vi "Configure Modulation(ASK).vi"(0 "VISA resource name":refnum<visa-resource-name>, 1 "Enable ASK Modulation (F: Disable)":bool, 2 "ASK Amplitude (0 Vpp)":dbl, 5 "Channel (1: Channel 1)":i32(ring)=1 items=["Channel 1"=1, "Channel 2"=2], 7 "ASK Source (0: Internal)":i32(ring) items=["Internal", "External"], 9 "Modulating Polarity (0: Positive)":i32(ring) items=["Positive", "Negative"], 11 "error in (no error)":errorcluster, 12 "Amplitude Unit (0: Vpp)":i32(ring) items=["Vpp", "Vrms", "dBm"], 13 "ASK Rate (100 Hz)":dbl=100.0) -> (4 "VISA resource name out":refnum<visa-resource-name>, 15 "error out":errorcluster)   [LabVIEW 2012, in "RIGOL DG4000 Series.lvlib"]
doc: "Configures ASK (Amplitude Shift Keying) modulation."
uses:
  <instrlib>/RIGOL DG4000 Series/RIGOL DG4000 Series.lvlib
panel:
  # "Amplitude Settings"
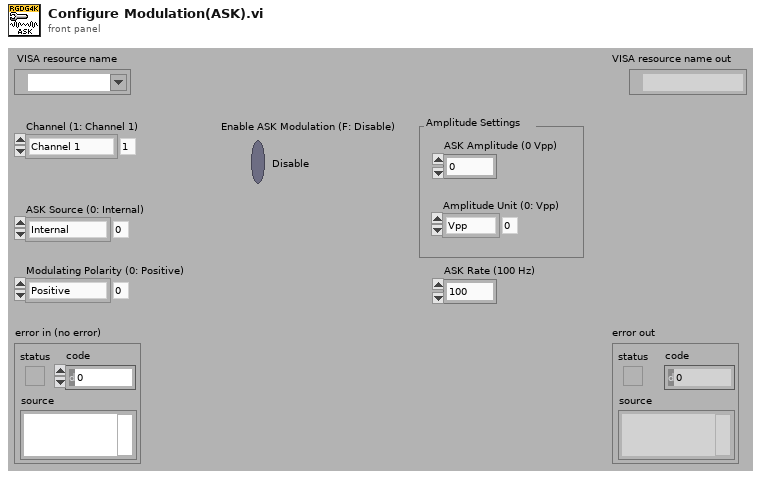
[diagram p1: front panel]
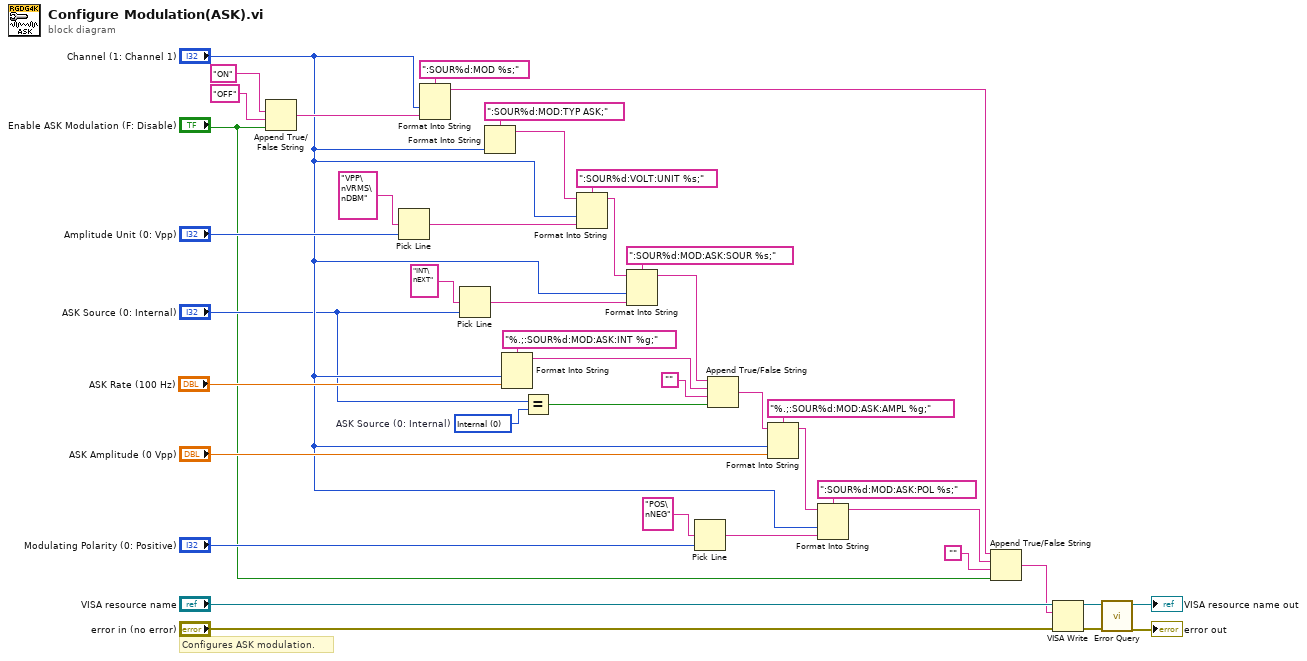
[diagram p0: block diagram]
diagram:
  w10 = 0 items=["Internal", "External"]  # ASK Source (0: Internal)
  # "Configures ASK modulation."
  n1 = Append True/False String(1:"Enable ASK Modulation (F: Disable)", 2:"OFF", 3:"ON") -> (0:w39:string)  [unwired: 1 out]
  n2 = Pick Line(multi-line string="VPP\nVRMS\nDBM", line index="Amplitude Unit (0: Vpp)") -> (output string=w33:string)  [unwired: 1 out]
  n3 = Format Into String(format string=":SOUR%d:MOD %s;", "Channel (1: Channel 1)", w39) -> (resulting string=w4:string)  [unwired: 2 in, 1 out]
  n4 = Pick Line(multi-line string="INT\nEXT", line index="ASK Source (0: Internal)") -> (output string=w29:string)  [unwired: 1 out]
  n5 = Format Into String(format string=":SOUR%d:MOD:TYP ASK;", "Channel (1: Channel 1)") -> (resulting string=w35:string)  [unwired: 2 in, 1 out]
  n6 = Format Into String(format string="%.;:SOUR%d:MOD:ASK:INT %g;", "Channel (1: Channel 1)", "ASK Rate (100 Hz)") -> (resulting string=w12:string)  [unwired: 2 in, 1 out]
  n7 = Equal?(x="ASK Source (0: Internal)", y=w10) -> (x = y?=w8:bool)
  n8 = Format Into String(format string=":SOUR%d:VOLT:UNIT %s;", initial string=w35, "Channel (1: Channel 1)", w33) -> (resulting string=w31:string)  [unwired: 1 in, 1 out]
  n9 = Format Into String(format string=":SOUR%d:MOD:ASK:SOUR %s;", initial string=w31, "Channel (1: Channel 1)", w29) -> (resulting string=w14:string)  [unwired: 1 in, 1 out]
  n10 = Pick Line(multi-line string="POS\nNEG", line index="Modulating Polarity (0: Positive)") -> (output string=w20:string)  [unwired: 1 out]
  n11 = Append True/False String(1:w8, 2:"", 3:w12, 4:w14) -> (0:w7:string)
  n12 = Format Into String(format string="%.;:SOUR%d:MOD:ASK:AMPL %g;", initial string=w7, "Channel (1: Channel 1)", "ASK Amplitude (0 Vpp)") -> (resulting string=w22:string)  [unwired: 1 in, 1 out]
  n13 = Format Into String(format string=":SOUR%d:MOD:ASK:POL %s;", initial string=w22, "Channel (1: Channel 1)", w20) -> (resulting string=w3:string)  [unwired: 1 in, 1 out]
  n14 = Append True/False String(1:"Enable ASK Modulation (F: Disable)", 2:"", 3:w3, 4:w4) -> (0:w1:string)
  n15 = VISA Write(VISA resource name="VISA resource name", write buffer=w1, error in (no error)="error in (no error)") -> (VISA resource name out=w17:refnum<visa-resource-name>, error out=w16:errorcluster)  [unwired: 1 out]
  n16 = call <instrlib>:"Error Query.vi"("error in (no error)"=w16, "VISA resource name"=w17) -> ("error out"=→"error out":errorcluster, "VISA resource name out"=→"VISA resource name out":refnum<visa-resource-name>)  [unwired: 8 out]
